vi "TEST_ASIC_MAJandADDS_NEW.vi"(5 "threshold":i32[][](array[numeric])=[[602, 520, 522, 602, 518, 602, 508], [518, 522, 524, 522, 520, 512, 510], [518, 524, 526, 522, 5262, 514, 514], [526, 530, 530, 528, 532, 520, 518], [564, 562, 556, 518, 562, 554, 546]], 7 "Serial Number":string="SN_143", 8 "error in (no error)":errorcluster, 11 "Instrument VISA in":T1={"AWG VISA"="AgilentGenerator1", "Oscilloscope  VISA "="AgilentOsciloscope", "Integration Board IP"="172.16.17.47", "connection ID"=refnum, "report out"=refnum, "report file path"=path "C:/Users/omartinez/Desktop/L0nL1_Results"}) -> (0 "error out":errorcluster, 3 "Instrument VISA out":T1={"AWG VISA"="AgilentGenerator1", "Oscilloscope  VISA "="AgilentOsciloscope", "Integration Board IP"="172.16.17.47", "connection ID"=refnum, "report out"=refnum, "report file path"=path "C:/Users/omartinez/Desktop/L0nL1_Results"})   [LabVIEW 2012]
uses:
  <vilib>/Utility/NIReport.llb/NI_report.lvclass
  <vilib>/Utility/NIReport.llb/HTML/NI_HTML.lvclass
  <instrlib>/Agilent 8000 Series/Public/Configure/Configure Math (Binary Operation).vi
  Sum_Abrilader/L0_Sum_Adder Folder/C/Program Files/National Instruments/LabVIEW 2012/instr.lib/Agilent 8000 Series/Public/Data/Low Level/Fetch Measurement (More).vi
  <instrlib>/Agilent 8000 Series/Agilent 8000 Series.lvlib
  Sum_Abrilader/L0_Sum_Adder Folder/C/Program Files/National Instruments/LabVIEW 2012/instr.lib/Agilent 81150/Agilent 81150.lvlib
panel:
  in  "Voltages comprobation":dbl[](array[numeric])=[0.05, 0.1, 0.2, 0.5, 0.8]
  in  "Channels \nCombinations":i32[](array[numeric])=[3, 12, 48, 96, 7, 28, 112, 15, 120, 31, 124, 63, 126, 127]
  in  "Voltages":dbl[](array[numeric])=[0.05, 0.1, 0.2, 0.5, 0.8]
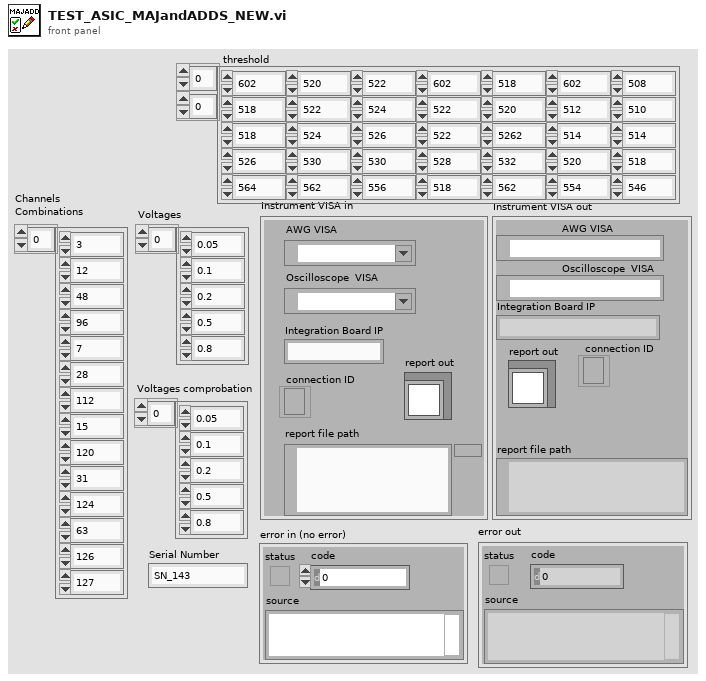
[diagram p1: front panel]
types:
  T1 = cluster{"AWG VISA":refnum<visa-resource-name>, "Oscilloscope  VISA ":refnum<visa-resource-name>, "Integration Board IP":string, "connection ID":refnum<k5>, "report out":refnum<class "NI_report.lvclass">, "report file path":path}
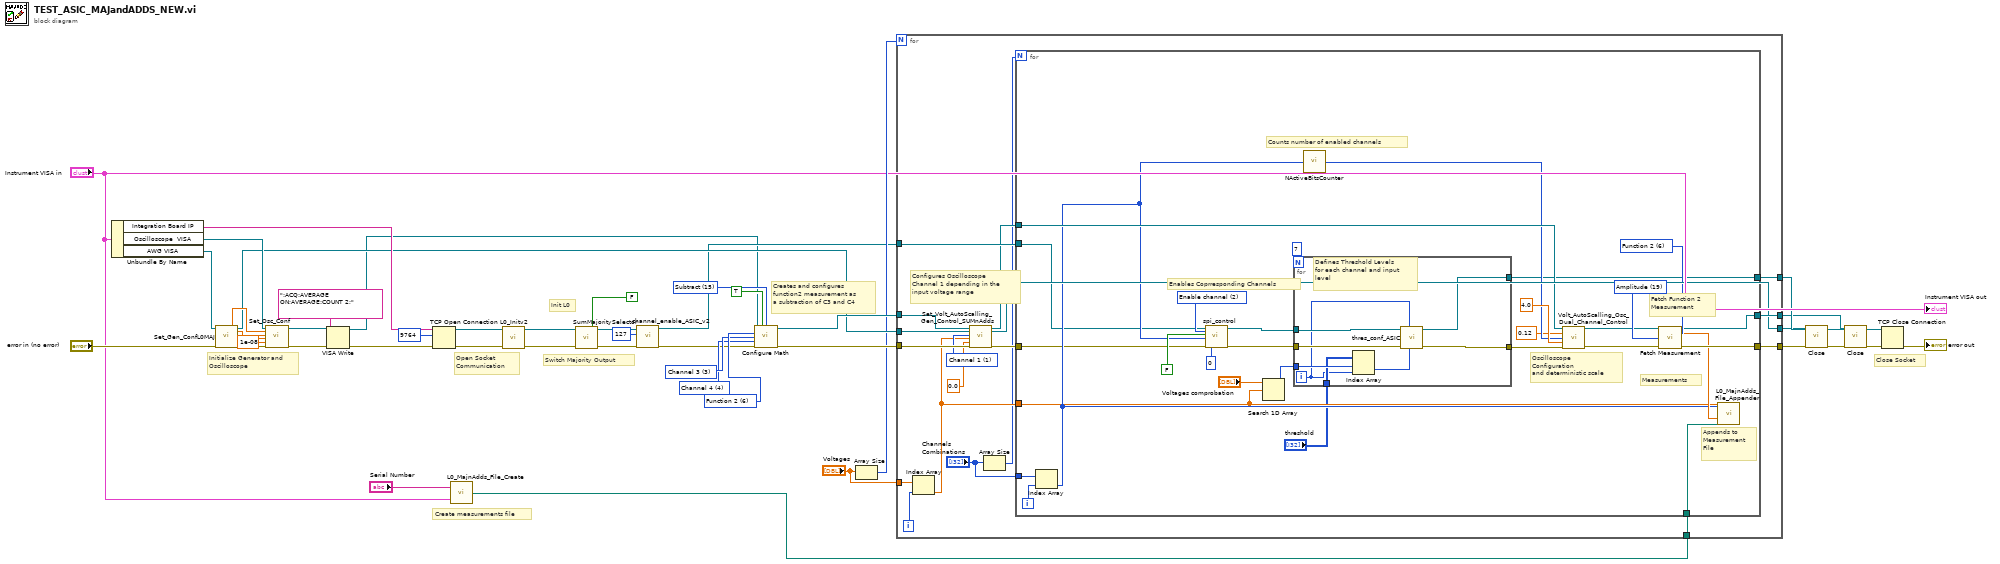
[diagram p0: block diagram]
diagram:
  w42 = u16 6 items=["Function 1"=5, "Function 2"=6, "Function 3"=7, "Function 4"=8] ("Math Channel (5: Function 1)")
  w43 = u16 15 items=["Add"=12, "Divide"=13, "Multiply"=14, "Subtract"=15, "Common Mode"=16, "Versus"=17] ("Math Operation (12: Add)")
  w41 = 3 items=["Channel 1"=1, "Channel 2"=2, "Channel 3"=3, "Channel 4"=4] ("Channel (1: Channel 1)")
  w40 = 4 items=["Channel 1"=1, "Channel 2"=2, "Channel 3"=3, "Channel 4"=4] ("Channel (1: Channel 1)")
  # "Close Socket"
  # "Create measurements file"
  # "Init L0"
  # "Switch Majority Output"
  # "Initialize Generator and \nOscilloscope"
  # "Creates and configures\nfunction2 measurement as\na subtraction of C3 and C4"
  # "Open Socket\nCommunication"
  n1 = Unbundle By Name("Instrument VISA in") -> ("Integration Board IP"=w38:string, "Oscilloscope  VISA"=w30:refnum<visa-resource-name>, "AWG VISA"=w31:refnum<visa-resource-name>)
  n2 = call "Set_Gen_ConfL0MAJ.vi"("AWG VISA"=w31, "error in (no error)"="error in (no error)") -> ("Amplitude 1 OUT"=w35:dbl, "VISA resource name out"=w29:refnum<visa-resource-name>, "Pulse Width in seconds 1 OUT"=w34:dbl, "Trigger Level 1"=w33:dbl, "error out"=w36:errorcluster)  [unwired: 10 in, 3 out]
  n3 = call "Set_Osc_Conf.vi"("VISA resource name"=w30, "Amplitude IN"=w35, "Trigger Level IN"=w33, "Pulse Width in seconds IN"=w34, "Position 1"=1e-08, "error in (no error)"=w36) -> ("VISA resource name out"=w7:refnum<visa-resource-name>, "error out"=w9:errorcluster)  [unwired: 12 in]
  n4 = VISA Write(VISA resource name=w7, write buffer=":ACQ:AVERAGE ON;AVERAGE:COUNT 2;", error in (no error)=w9) -> (VISA resource name out=w6:refnum<visa-resource-name>, error out=w8:errorcluster)  [unwired: 1 out]
  n5 = TCP Open Connection(address=w38, remote port or service name=u16 9764, error in (no error)=w8) -> (connection ID=w18:refnum<k5>, error out=w19:errorcluster)  [unwired: 2 in]
  n6 = call "L0_MajnAdds_File_Create.vi"("input cluster"="Instrument VISA in", "Serial Number"="Serial Number") -> ("appended path"=w23:path)
  n7 = call "L0_Initv2.vi"("error in"=w19, "connection ID in"=w18) -> ("error out"=w22:errorcluster, "connection ID out"=w21:refnum<k5>)  [unwired: 8 in]
  n8 = call "SumMajoritySelector.vi"("On Sum\nOff Majority"=FALSE ("On Sum\nOff Majority"), "error in (no error)"=w22, "connection ID"=w21) -> ("error out"=w15:errorcluster, "connection ID out"=w13:refnum<k5>)  [unwired: 5 in]
  n9 = call "channel_enable_ASIC_v2.vi"("error in"=w15, "Channel Combination"=u32 127, "Connection ID in"=w13) -> ("error out"=w14:errorcluster, "Connection ID out"=w12:refnum<k5>)  [unwired: 7 in]
  n10 = call-poly <instrlib>:"Configure Math.vi"("VISA resource name"=w6, "Enable Math Channel (T:Enable)"=TRUE, "Math Operation (12: Add)"=w43, "Math Channel (5: Function 1)"=w42, "Math Operand (1: Channel 1)"=w41, "Math Operand (2: Channel 2)"=w40, "error in (no error)"=w14) -> ("VISA resource name out"=w37:refnum<visa-resource-name>, "error out"=w39:errorcluster)  [unwired: 7 in]
  n11 = Array Size(array="Voltages") -> (size(s)=w27:i32)
  n12 = for {
    N: w27 -> [_]
    tunnel: w39 -> [w63]
    tunnel: w12 -> [w62]
    tunnel: [w61] -> w4
    tunnel: w37 -> [w60]
    tunnel: w29 -> [w59]
    tunnel: "Voltages" -> [w54]
    tunnel: w23 -> [w49]
    tunnel: [w48] -> w16
    tunnel: [w47] -> w2
    tunnel: [w46] -> w1
    i -> [w53]
    w58 = 1 items=["Channel 1"=1, "Channel 2"=2, "Channel 3"=3, "Channel 4"=4] ("Channel")
    # "Configures Oscilloscope\nChannel 1 depending in the \ninput voltage range"
    n13 = Index Array(array=w54, index=w53) -> (element=w52:dbl)
    n14 = call "Set_Volt_AutoScalling_Gen_Control_SUMnAdds.vi"("VISA Oscilloscope"=w60, "VISA Generator"=w59, "Channel"=w58, "Amplitude"=w52, "DC Offset"=0.0, "error in (no error)"=w63) -> ("VISA Oscilloscope"=w55:refnum<visa-resource-name>, "VISA Generator"=w46:refnum<visa-resource-name>, "error out"=w56:errorcluster)  [unwired: 11 in]
    n15 = Array Size(array="Channels \nCombinations") -> (size(s)=w50:i32)
    n16 = for {
      N: w50 -> [_]
      tunnel: w62 -> [w65]
      tunnel: [w81] -> w61
      tunnel: w56 -> [w66]
      tunnel: w55 -> [w92]
      tunnel: w52 -> [w75]
      tunnel: "Channels \nCombinations" -> [w86]
      tunnel: w49 -> [w78]
      tunnel: [w71] -> w48
      tunnel: [w64] -> w47
      i -> [w85]
      w84 = 19 items=["Rise Time", "Fall Time", "Frequency", "Period", "Voltage RMS(AC)", "Voltage RMS(DC)", "Voltage RMS (AC,cycle)", "Voltage RMS (DC,cycle)", "Voltage Max", "Voltage Min", "Voltage Middle", "Voltage Vpp", "Voltage High", "Voltage Low", "Voltage Average", "Voltage Average (cycle)", "Width Negative", "Width Positive", "Duty Cycle Positive", "Amplitude", "Overshoot", "Preshoot", "Voltage Base", "Voltage Upper", "Time Max", "Time Min", "Color Grade Crossing", "Color Grade Eye Width", "Color Grade Eye Height", "Color Grade Eye Q-Factory", "Color Grade Eye Duty Cycle Distortion(Percent)", "Color Grade Eye Duty Cycle Distortion(Time)", "Color Grade Eye Jitter(PP)", "Color Grade Eye Width(RMS)", "Cycle-cycle Duty Jitter(Rising)", "Cycle-cycle Duty Jitter(Falling)", "Cycle-cycle Jitter(Rising)", "Cycle-cycle Jitter(Falling)", "Cycle-cycle - Width", "Cycle-cycle + Width", "Date Rate", "Unit Interval", "FFT Delta Frequency", "FFT Delta Magnitude", "FFT Frequency", "FFT Magnitude", "Slew Rate", "Area (Entire Display)", "Area(Single Cycle)", "Duty Cycle (Rising)", "Duty Cycle (Falling)"] ("Measurement Function (0: Rise Time)")
      w83 = 6 items=["Channel 1"=1, "Channel 2"=2, "Channel 3"=3, "Channel 4"=4, "Function 1"=5, "Function 2"=6, "Function 3"=7, "Function 4"=8, "Memory 1"=9, "Memory 2"=10, "Memory 3"=11, "Memory 4"=12] ("Channel (1: Channel 1)")
      w89 = u16 2 items=["Attenuation", "Clipping", "Enable channel", "Delay line", "ASIC"] ("Device")
      # "Appends to\nMeasurement\nFile"
      # "Counts number of enabled channels"
      # "Fetch Function 2\nMeasurement"
      # "Measurements"
      # "Enables Coprresponding Channels"
      # "Oscilloscope Configuration \nand deterministic scale"
      n17 = Index Array(array=w86, index=w85) -> (element=w77:i32)
      n18 = call "spi_control.vi"("connection ID"=w65, "Device"=w89, "Read/#write"=FALSE, "Data"=w77, "error in"=w66, "Id in"=0) -> ("connection ID out"=w68:refnum<k5>, "error out 2"=w67:errorcluster)  [unwired: 6 in, 6 out]
      n19 = Search 1D Array(1D array="Voltages comprobation", element=w75) -> (index of element=w74:i32)  [unwired: 1 in]
      n20 = for {
        N: 7 -> [_]
        tunnel: w74 -> [w99]
        tunnel: w67 -> [w100]
        tunnel: w68 -> [w97]
        tunnel: [w94] -> w72
        tunnel: [w93] -> w71
        tunnel: "threshold" -> [w96]
        i -> [w95]
        # "Defines Threshold Levels\nfor each channel and input\nlevel"
        n21 = Index Array(array=w96, index (row)=w99, index (col)=w95) -> (element=w98:i32)
        n22 = call "thres_conf_ASIC.vi"("threshold"=w98, "Ring"=w95, "error out 3"=w100, "connection ID"=w97) -> ("error out 2"=w94:errorcluster, "connection ID out"=w93:refnum<k5>)  [unwired: 4 in, 2 out]
      }
      n23 = call "NActiveBitsCounter.vi"("Input Number"=w77) -> ("N High Bits"=w87:i32)
      n24 = call "Volt_AutoScalling_Osc_Dual_Channel_Control.vi"("VISA Oscilloscope"=w92, "Voltage In"=0.12, "N Channels"=w87, "Offset Divider"=4.0, "error in"=w72) -> ("VISA resource name out"=w80:refnum<visa-resource-name>, "error out"=w82:errorcluster)  [unwired: 9 in]
      n25 = call-poly "Fetch Measurement.vi"("VISA resource name"=w80, "Channel (1: Channel 1)"=w83, "Measurement Function (0: Rise Time)"=w84, "error in (no error)"=w82) -> ("VISA resource name out"=w64:refnum<visa-resource-name>, "Measurement"=w79:dbl, "error out"=w81:errorcluster)  [unwired: 9 in]
      n26 = call "L0_MajnAdds_File_Appender.vi"("Vin"=w75, "CH"=w77, "Vmeas"=w79, "file path (dialog if empty)"=w78) -> ()  [unwired: 24 in]
    }
  }
  n27 = call <instrlib>:"Close.vi"("error in (no error)"=w4, "VISA resource name"=w1) -> ("error out"=w5:errorcluster)  [unwired: 9 in]
  n28 = call <instrlib>:"Close.vi"("error in (no error)"=w5, "VISA resource name"=w2) -> ("error out"=w3:errorcluster)  [unwired: 9 in]
  n29 = TCP Close Connection(connection ID=w16, error in (no error)=w3) -> (error out=→"error out":errorcluster)  [unwired: 1 in, 1 out]
  "Instrument VISA out" <- "Instrument VISA in"
